vi "XYZ Points generator.vi"(5 "Symmetric":bool, 10 "Number of points":i32=3 min=3 step=2, 11 "FOV/ Z-range":dbl) -> (2 "Normalised centre Points":dbl[](array[numeric]), 3 "Stage Points":dbl[](array[numeric]))   [LabVIEW 2020]
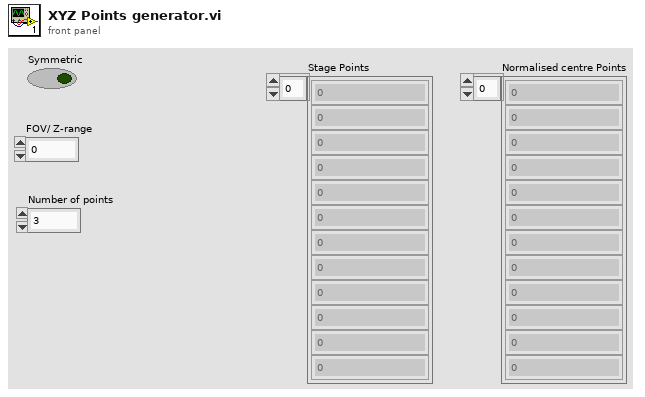
[diagram p1: front panel]
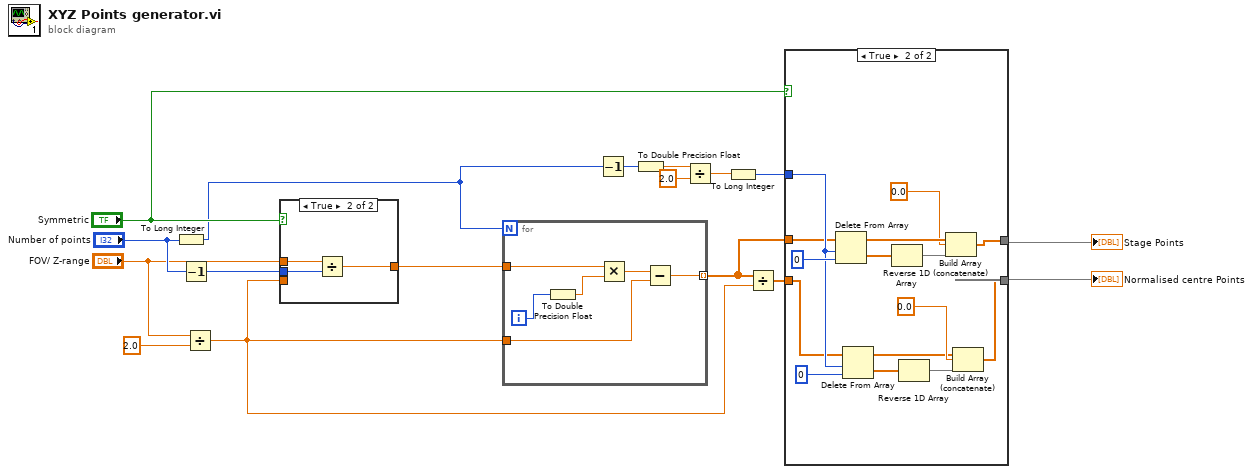
[diagram p0: block diagram]
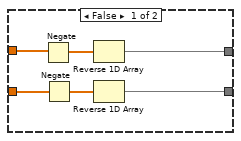
[diagram p2: hidden frame]
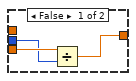
[diagram p3: hidden frame]
diagram:
  n1 = To Long Integer(number="Number of points") -> (32bit integer=w6:i32)
  n2 = Decrement(x="Number of points") -> (x-1=w13:i32)
  n3 = Divide(x="FOV/ Z-range", y=2.0) -> (x/y=w12:dbl)
  n4 = case shown="True" "Symmetric" {
    tunnel: "FOV/ Z-range" -> [_ w23]
    tunnel: [w18 w22] -> w14
    tunnel: w13 -> [w19 w21]
    tunnel: w12 -> [w20 _]
    frame False {
      n5 = Divide(x=w20, y=w19) -> (x/y=w18:dbl)
    }
    frame True {
      n6 = Divide(x=w23, y=w21) -> (x/y=w22:dbl)
    }
  }
  n7 = for {
    N: w6 -> [_]
    tunnel: w14 -> [w29]
    tunnel: w12 -> [w25]
    tunnel: [w24] -> w9 mode=indexing
    i -> [w28]
    n8 = To Double Precision Float(number=w28) -> (double precision float=w27:dbl)
    n9 = Multiply(x=w29, y=w27) -> (x*y=w26:dbl)
    n10 = Subtract(x=w26, y=w25) -> (x-y=w24:dbl)
  }
  n11 = Decrement(x=w6) -> (x-1=w5:i32)
  n12 = To Double Precision Float(number=w5) -> (double precision float=w4:dbl)
  n13 = Divide(x=w4, y=2.0) -> (x/y=w2:dbl)
  n14 = To Long Integer(number=w2) -> (32bit integer=w1:i32)
  n15 = Divide(x=w9, y=w12) -> (x/y=w10:dbl[])
  n16 = case shown="True" "Symmetric" {
    tunnel: w10 -> [w34 w36]
    tunnel: w9 -> [w35 w38]
    tunnel: [w31 w45] -> w8
    tunnel: [w30 w37] -> w7
    tunnel: w1 -> [_ w39]
    frame False {
      n17 = Negate(x=w35) -> (-x=w33:dbl[])
      n18 = Negate(x=w34) -> (-x=w32:dbl[])
      n19 = Reverse 1D Array(array=w33) -> (reversed array=w31:dbl[])
      n20 = Reverse 1D Array(array=w32) -> (reversed array=w30:dbl[])
    }
    frame True {
      n21 = Delete From Array(array=w38, length=w39, index=0) -> (deleted portion=w49:dbl[], array with subset deleted=w48:dbl[])
      n22 = Delete From Array(array=w36, length=w39, index=0) -> (deleted portion=w41:dbl[], array with subset deleted=w42:dbl[])
      n23 = Reverse 1D Array(array=w49) -> (reversed array=w46:dbl[])
      n24 = Reverse 1D Array(array=w41) -> (reversed array=w44:dbl[])
      n25 = Build Array (concatenate)(w48, 0.0, w46) -> (w45:dbl[])
      n26 = Build Array (concatenate)(w42, 0.0, w44) -> (w37:dbl[])
    }
  }
  "Stage Points" <- w8
  "Normalised centre Points" <- w7
